vi "triquimejorado.vi"() -> ()   [LabVIEW 2021]
panel:
  out "appended array":u16[][](array[numeric])
  in  "OK Button":bool
  in  "x":bool
  in  "Ring 9":u16(ring)
  in  "Ring 8":u16(ring)
  in  "Ring 6":u16(ring)
  in  "Ring 5":u16(ring)
  in  "Ring 7":u16(ring)
  in  "Ring 4":u16(ring)
  in  "Ring 3":u16(ring)
  in  "Ring 2":u16(ring)
  in  "Ring":u16(ring)
  # "0"
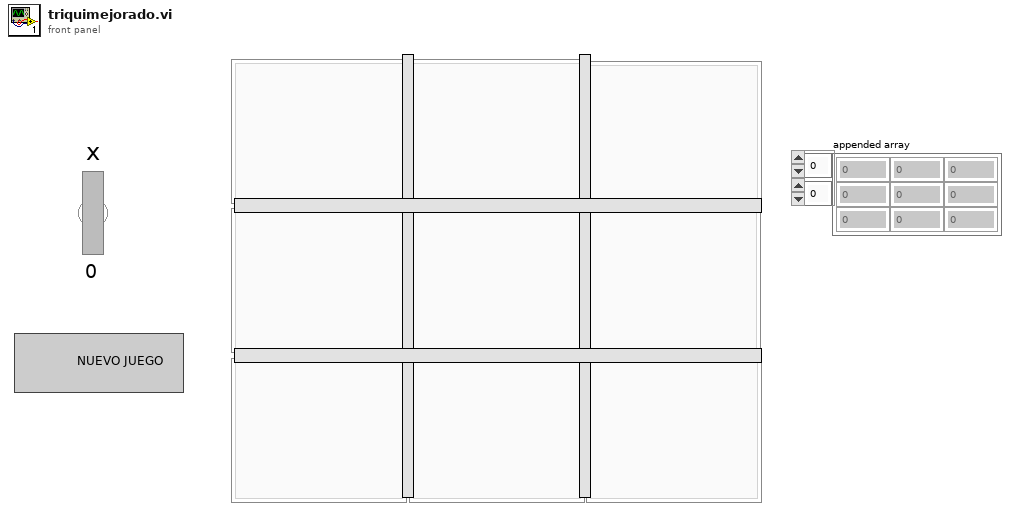
[diagram p1: front panel]
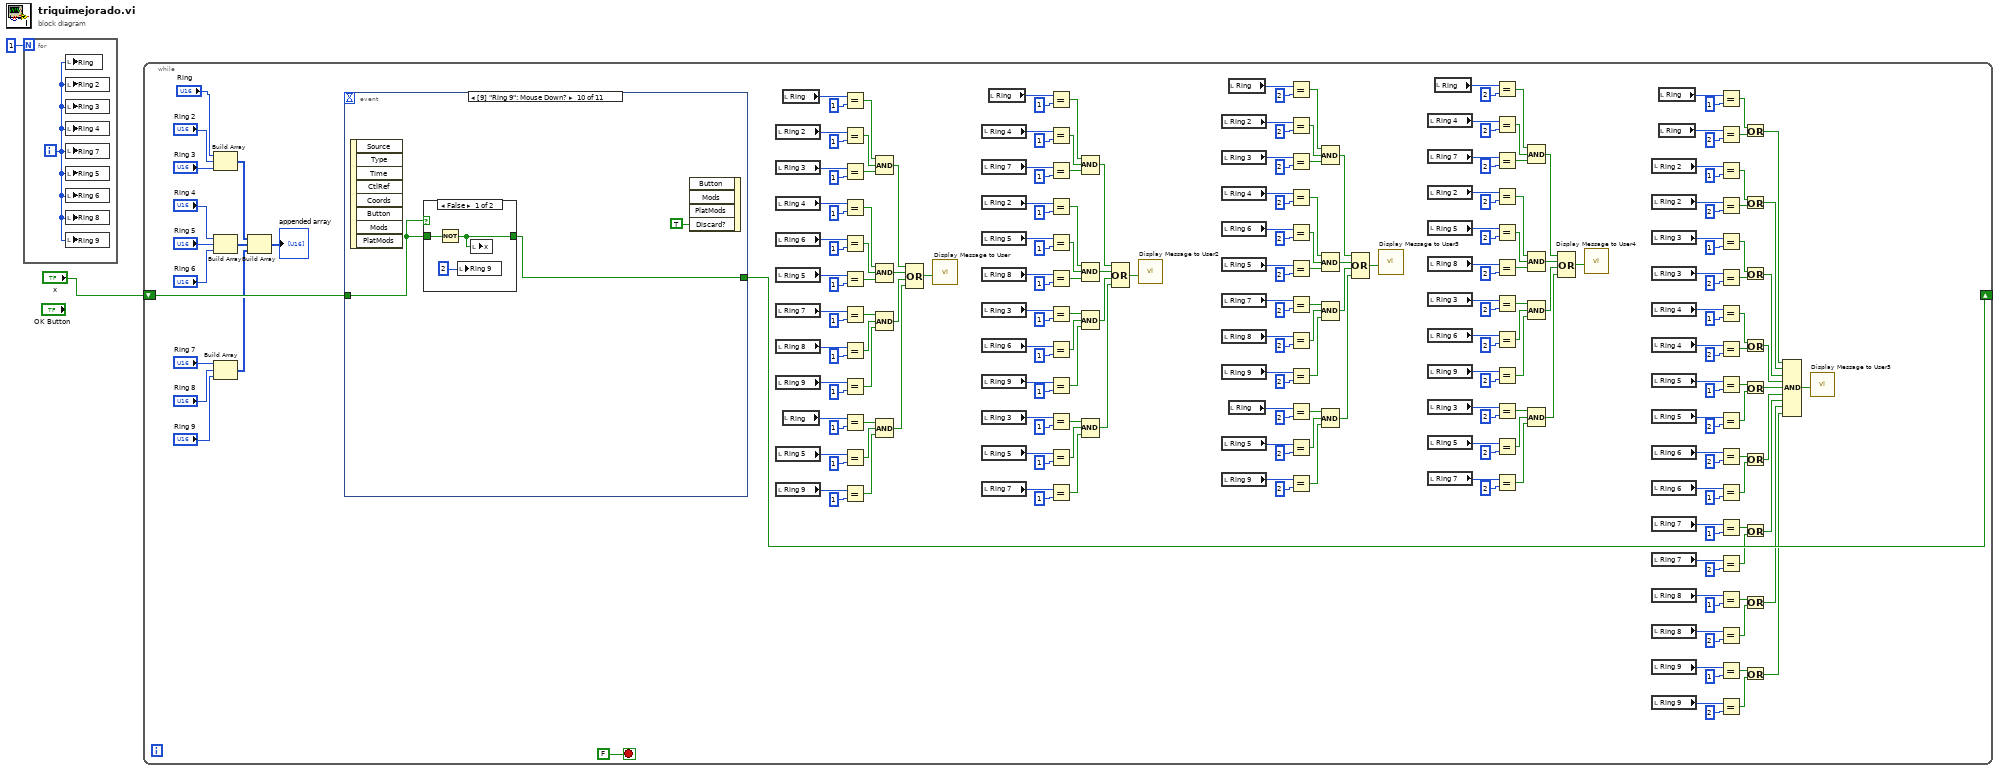
[diagram p0: block diagram]
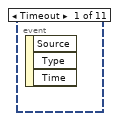
[diagram p2: hidden frame]
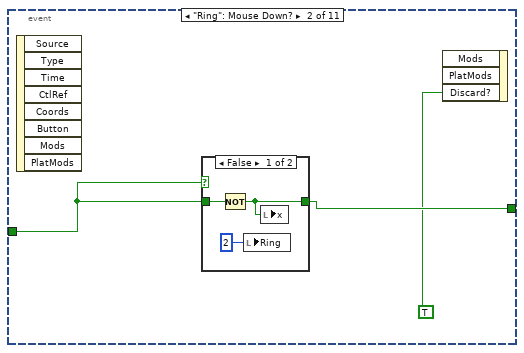
[diagram p3: hidden frame]
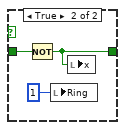
[diagram p4: hidden frame]
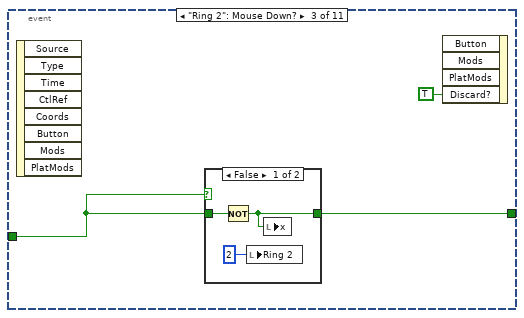
[diagram p5: hidden frame]
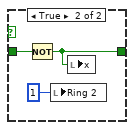
[diagram p6: hidden frame]
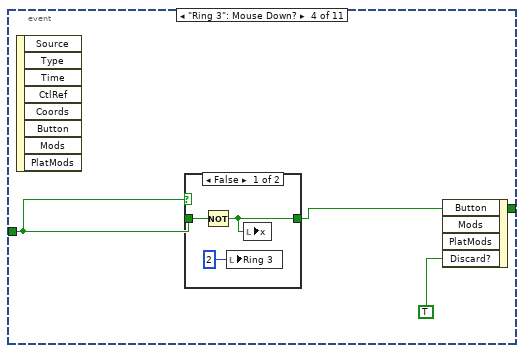
[diagram p7: hidden frame]
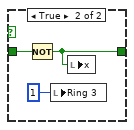
[diagram p8: hidden frame]
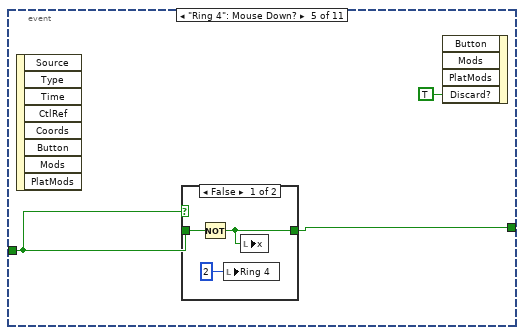
[diagram p9: hidden frame]
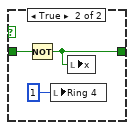
[diagram p10: hidden frame]
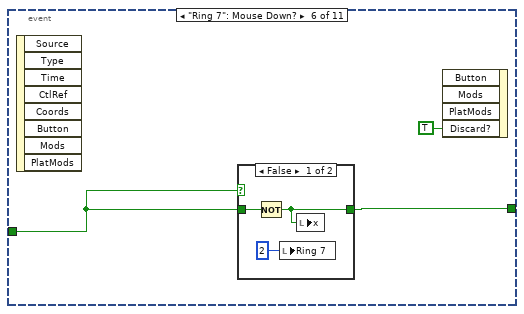
[diagram p11: hidden frame]
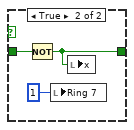
[diagram p12: hidden frame]
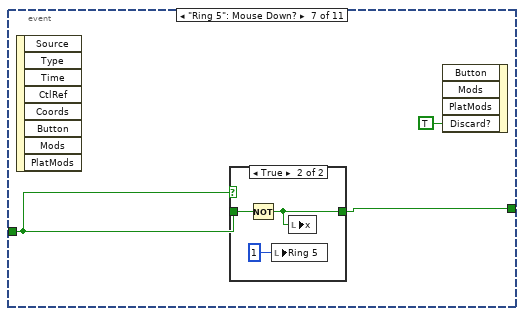
[diagram p13: hidden frame]
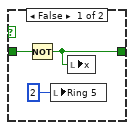
[diagram p14: hidden frame]
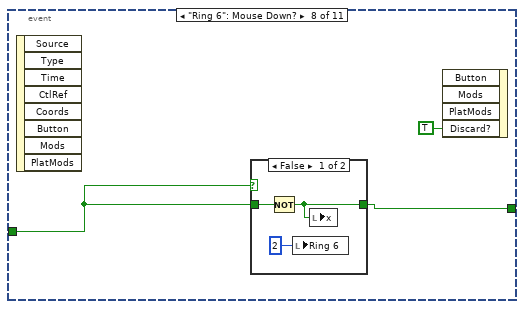
[diagram p15: hidden frame]
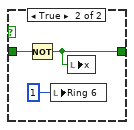
[diagram p16: hidden frame]
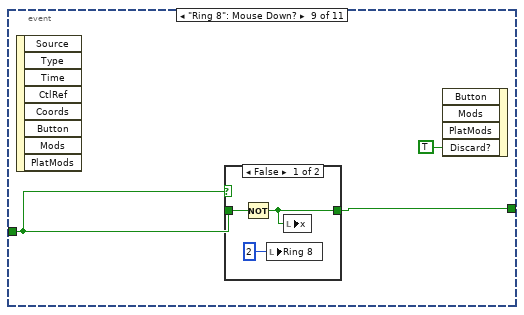
[diagram p17: hidden frame]
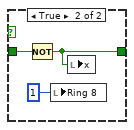
[diagram p18: hidden frame]
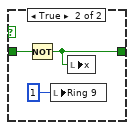
[diagram p19: hidden frame]
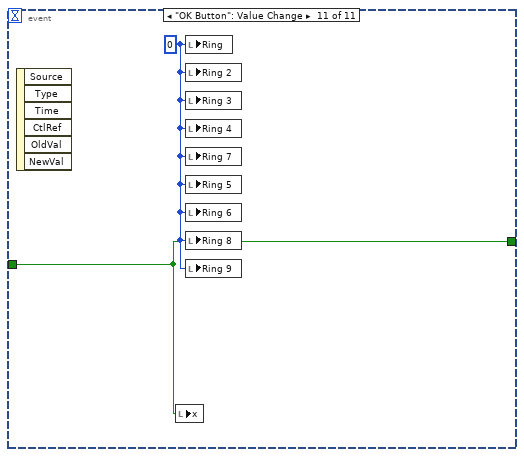
[diagram p20: hidden frame]
diagram:
  n1 = for {
    N: 1 -> [_]
    i -> [w3]
    n2 = local write "Ring"(w3) -> ()
    n3 = local write "Ring 2"(w3) -> ()
    n4 = local write "Ring 3"(w3) -> ()
    n5 = local write "Ring 4"(w3) -> ()
    n6 = local write "Ring 7"(w3) -> ()
    n7 = local write "Ring 5"(w3) -> ()
    n8 = local write "Ring 6"(w3) -> ()
    n9 = local write "Ring 8"(w3) -> ()
    n10 = local write "Ring 9"(w3) -> ()
  }
  n11 = while {
    shift-right: [w247] -> _
    shift-left: "x" -> [w246]
    stop <- FALSE stop-if-true
    n12 = Build Array("Ring", "Ring 2", "Ring 3") -> (w75:u16[])
    n13 = Build Array("Ring 4", "Ring 5", "Ring 6") -> (w74:u16[])
    n14 = Build Array("Ring 7", "Ring 8", "Ring 9") -> (w76:u16[])
    n15 = Build Array(w75, w74, w76) -> (→"appended array":u16[][])
    n16 = event shown="[9] \"Ring 9\": Mouse Down?" {
      selector: _ -> [_ _ _ _ _ _ _ _ _ _ _]
      dyn-events: _ -> [_ _ _ _ _ _ _ _ _ _ _]
      timeout: _ -> [_ _ _ _ _ _ _ _ _ _ _]
      tunnel: [_ w250 w258 w267 w276 w286 w295 w304 w312 w321 w329] -> w247
      tunnel: w246 -> [_ w248 w259 w268 w277 w285 w294 w303 w313 w322 w329]
      event Timeout {
        n17 = event-data() -> ()  [unwired: 1 in, 3 out]
      }
      event "Ring": Mouse Down? {
        n18 = event-data() -> ()  [unwired: 1 in, 8 out]
        n19 = case shown="False" w248 {
          tunnel: [w252 w255] -> w250
          tunnel: w248 -> [w251 w254]
          frame False {
            n20 = Not(x=w251) -> (.not. x?=w252:bool)
            n21 = local write "Ring"(u16 2 ("Ring")) -> ()
            n22 = local write "x"(w252) -> ()
          }
          frame True {
            n23 = Not(x=w254) -> (.not. x?=w255:bool)
            n24 = local write "Ring"(u16 1 ("Ring")) -> ()
            n25 = local write "x"(w255) -> ()
          }
        }
        n26 = event-data("Discard?"=TRUE) -> ()  [unwired: 3 in, 1 out]
      }
      event "Ring 2": Mouse Down? {
        n27 = event-data() -> ()  [unwired: 1 in, 8 out]
        n28 = case shown="False" w259 {
          tunnel: w259 -> [w261 w264]
          tunnel: [w260 w263] -> w258
          frame False {
            n29 = Not(x=w261) -> (.not. x?=w260:bool)
            n30 = local write "Ring 2"(u16 2 ("Ring 2")) -> ()
            n31 = local write "x"(w260) -> ()
          }
          frame True {
            n32 = Not(x=w264) -> (.not. x?=w263:bool)
            n33 = local write "Ring 2"(u16 1 ("Ring 2")) -> ()
            n34 = local write "x"(w263) -> ()
          }
        }
        n35 = event-data("Discard?"=TRUE) -> ()  [unwired: 4 in, 1 out]
      }
      event "Ring 3": Mouse Down? {
        n36 = event-data() -> ()  [unwired: 1 in, 8 out]
        n37 = case shown="False" w268 {
          tunnel: w268 -> [w270 w273]
          tunnel: [w269 w272] -> w267
          frame False {
            n38 = Not(x=w270) -> (.not. x?=w269:bool)
            n39 = local write "Ring 3"(u16 2 ("Ring 2")) -> ()
            n40 = local write "x"(w269) -> ()
          }
          frame True {
            n41 = Not(x=w273) -> (.not. x?=w272:bool)
            n42 = local write "Ring 3"(u16 1 ("Ring 2")) -> ()
            n43 = local write "x"(w272) -> ()
          }
        }
        n44 = event-data("Discard?"=TRUE) -> ()  [unwired: 4 in, 1 out]
      }
      event "Ring 4": Mouse Down? {
        n45 = event-data() -> ()  [unwired: 1 in, 8 out]
        n46 = case shown="False" w277 {
          tunnel: w277 -> [w279 w282]
          tunnel: [w278 w281] -> w276
          frame False {
            n47 = Not(x=w279) -> (.not. x?=w278:bool)
            n48 = local write "Ring 4"(u16 2 ("Ring 2")) -> ()
            n49 = local write "x"(w278) -> ()
          }
          frame True {
            n50 = Not(x=w282) -> (.not. x?=w281:bool)
            n51 = local write "Ring 4"(u16 1 ("Ring 2")) -> ()
            n52 = local write "x"(w281) -> ()
          }
        }
        n53 = event-data("Discard?"=TRUE) -> ()  [unwired: 4 in, 1 out]
      }
      event "Ring 7": Mouse Down? {
        n54 = event-data() -> ()  [unwired: 1 in, 8 out]
        n55 = case shown="False" w285 {
          tunnel: w285 -> [w288 w291]
          tunnel: [w287 w290] -> w286
          frame False {
            n56 = Not(x=w288) -> (.not. x?=w287:bool)
            n57 = local write "Ring 7"(u16 2 ("Ring 2")) -> ()
            n58 = local write "x"(w287) -> ()
          }
          frame True {
            n59 = Not(x=w291) -> (.not. x?=w290:bool)
            n60 = local write "Ring 7"(u16 1 ("Ring 2")) -> ()
            n61 = local write "x"(w290) -> ()
          }
        }
        n62 = event-data("Discard?"=TRUE) -> ()  [unwired: 4 in, 1 out]
      }
      event "Ring 5": Mouse Down? {
        n63 = event-data() -> ()  [unwired: 1 in, 8 out]
        n64 = case shown="True" w294 {
          tunnel: w294 -> [w297 w300]
          tunnel: [w296 w299] -> w295
          frame False {
            n65 = Not(x=w297) -> (.not. x?=w296:bool)
            n66 = local write "Ring 5"(u16 2 ("Ring 2")) -> ()
            n67 = local write "x"(w296) -> ()
          }
          frame True {
            n68 = Not(x=w300) -> (.not. x?=w299:bool)
            n69 = local write "Ring 5"(u16 1 ("Ring 2")) -> ()
            n70 = local write "x"(w299) -> ()
          }
        }
        n71 = event-data("Discard?"=TRUE) -> ()  [unwired: 4 in, 1 out]
      }
      event "Ring 6": Mouse Down? {
        n72 = event-data() -> ()  [unwired: 1 in, 8 out]
        n73 = case shown="False" w303 {
          tunnel: w303 -> [w306 w309]
          tunnel: [w305 w308] -> w304
          frame False {
            n74 = Not(x=w306) -> (.not. x?=w305:bool)
            n75 = local write "Ring 6"(u16 2 ("Ring 2")) -> ()
            n76 = local write "x"(w305) -> ()
          }
          frame True {
            n77 = Not(x=w309) -> (.not. x?=w308:bool)
            n78 = local write "Ring 6"(u16 1 ("Ring 2")) -> ()
            n79 = local write "x"(w308) -> ()
          }
        }
        n80 = event-data("Discard?"=TRUE) -> ()  [unwired: 4 in, 1 out]
      }
      event "Ring 8": Mouse Down? {
        n81 = event-data() -> ()  [unwired: 1 in, 8 out]
        n82 = case shown="False" w313 {
          tunnel: w313 -> [w315 w318]
          tunnel: [w314 w317] -> w312
          frame False {
            n83 = Not(x=w315) -> (.not. x?=w314:bool)
            n84 = local write "Ring 8"(u16 2 ("Ring 2")) -> ()
            n85 = local write "x"(w314) -> ()
          }
          frame True {
            n86 = Not(x=w318) -> (.not. x?=w317:bool)
            n87 = local write "Ring 8"(u16 1 ("Ring 2")) -> ()
            n88 = local write "x"(w317) -> ()
          }
        }
        n89 = event-data("Discard?"=TRUE) -> ()  [unwired: 4 in, 1 out]
      }
      event "Ring 9": Mouse Down? {
        n90 = event-data() -> ()  [unwired: 1 in, 8 out]
        n91 = case shown="False" w322 {
          tunnel: w322 -> [w324 w327]
          tunnel: [w323 w326] -> w321
          frame False {
            n92 = Not(x=w324) -> (.not. x?=w323:bool)
            n93 = local write "Ring 9"(u16 2 ("Ring 2")) -> ()
            n94 = local write "x"(w323) -> ()
          }
          frame True {
            n95 = Not(x=w327) -> (.not. x?=w326:bool)
            n96 = local write "Ring 9"(u16 1 ("Ring 2")) -> ()
            n97 = local write "x"(w326) -> ()
          }
        }
        n98 = event-data("Discard?"=TRUE) -> ()  [unwired: 4 in, 1 out]
      }
      event "OK Button": Value Change {
        w330 = u16 0 ("Ring")
        n99 = event-data() -> ()  [unwired: 1 in, 6 out]
        n100 = local write "x"(w329) -> ()
        n101 = local write "Ring"(w330) -> ()
        n102 = local write "Ring 2"(w330) -> ()
        n103 = local write "Ring 3"(w330) -> ()
        n104 = local write "Ring 4"(w330) -> ()
        n105 = local write "Ring 7"(w330) -> ()
        n106 = local write "Ring 5"(w330) -> ()
        n107 = local write "Ring 6"(w330) -> ()
        n108 = local write "Ring 8"(w330) -> ()
        n109 = local write "Ring 9"(w330) -> ()
      }
    }
    n110 = local read "Ring 2"() -> (w243:u16)
    n111 = local read "Ring 3"() -> (w241:u16)
    n112 = local read "Ring 4"() -> (w230:u16)
    n113 = local read "Ring 6"() -> (w229:u16)
    n114 = local read "Ring 5"() -> (w228:u16)
    n115 = local read "Ring 7"() -> (w221:u16)
    n116 = local read "Ring 8"() -> (w220:u16)
    n117 = local read "Ring 9"() -> (w219:u16)
    n118 = local read "Ring 5"() -> (w213:u16)
    n119 = local read "Ring 9"() -> (w214:u16)
    n120 = local read "Ring"() -> (w245:u16)
    n121 = local read "Ring"() -> (w212:u16)
    n122 = Equal?(x=w245, y=u16 1) -> (x = y?=w239:bool)
    n123 = Equal?(x=w243, y=u16 1) -> (x = y?=w238:bool)
    n124 = Equal?(x=w241, y=u16 1) -> (x = y?=w237:bool)
    n125 = Equal?(x=w230, y=u16 1) -> (x = y?=w234:bool)
    n126 = Equal?(x=w229, y=u16 1) -> (x = y?=w235:bool)
    n127 = Equal?(x=w228, y=u16 1) -> (x = y?=w236:bool)
    n128 = Equal?(x=w221, y=u16 1) -> (x = y?=w224:bool)
    n129 = Equal?(x=w220, y=u16 1) -> (x = y?=w223:bool)
    n130 = Equal?(x=w219, y=u16 1) -> (x = y?=w222:bool)
    n131 = Equal?(x=w212, y=u16 1) -> (x = y?=w209:bool)
    n132 = Equal?(x=w213, y=u16 1) -> (x = y?=w210:bool)
    n133 = Equal?(x=w214, y=u16 1) -> (x = y?=w211:bool)
    n134 = Compound Arithmetic op=AND(w239, w238, w237) -> (w218:bool)
    n135 = Compound Arithmetic op=AND(w234, w235, w236) -> (w217:bool)
    n136 = Compound Arithmetic op=AND(w224, w223, w222) -> (w216:bool)
    n137 = Compound Arithmetic op=AND(w209, w210, w211) -> (w205:bool)
    n138 = Compound Arithmetic op=OR(w218, w217, w216, w205) -> (w215:bool)
    n139 = call "Display Message to User"("Enable"=w215) -> ()  [unwired: 9 in, 2 out]
    n140 = local read "Ring 4"() -> (w166:u16)
    n141 = local read "Ring 7"() -> (w168:u16)
    n142 = local read "Ring 2"() -> (w179:u16)
    n143 = local read "Ring 5"() -> (w180:u16)
    n144 = local read "Ring 8"() -> (w181:u16)
    n145 = local read "Ring 3"() -> (w188:u16)
    n146 = local read "Ring 6"() -> (w189:u16)
    n147 = local read "Ring 9"() -> (w190:u16)
    n148 = local read "Ring 3"() -> (w197:u16)
    n149 = local read "Ring 5"() -> (w196:u16)
    n150 = local read "Ring 7"() -> (w195:u16)
    n151 = local read "Ring"() -> (w164:u16)
    n152 = Equal?(x=w164, y=u16 1) -> (x = y?=w170:bool)
    n153 = Equal?(x=w166, y=u16 1) -> (x = y?=w171:bool)
    n154 = Equal?(x=w168, y=u16 1) -> (x = y?=w172:bool)
    n155 = Equal?(x=w179, y=u16 1) -> (x = y?=w175:bool)
    n156 = Equal?(x=w180, y=u16 1) -> (x = y?=w174:bool)
    n157 = Equal?(x=w181, y=u16 1) -> (x = y?=w173:bool)
    n158 = Equal?(x=w188, y=u16 1) -> (x = y?=w185:bool)
    n159 = Equal?(x=w189, y=u16 1) -> (x = y?=w186:bool)
    n160 = Equal?(x=w190, y=u16 1) -> (x = y?=w187:bool)
    n161 = Equal?(x=w197, y=u16 1) -> (x = y?=w200:bool)
    n162 = Equal?(x=w196, y=u16 1) -> (x = y?=w199:bool)
    n163 = Equal?(x=w195, y=u16 1) -> (x = y?=w198:bool)
    n164 = Compound Arithmetic op=AND(w170, w171, w172) -> (w191:bool)
    n165 = Compound Arithmetic op=AND(w175, w174, w173) -> (w192:bool)
    n166 = Compound Arithmetic op=AND(w185, w186, w187) -> (w193:bool)
    n167 = Compound Arithmetic op=AND(w200, w199, w198) -> (w204:bool)
    n168 = Compound Arithmetic op=OR(w191, w192, w193, w204) -> (w194:bool)
    n169 = call "Display Message to User2"("Enable"=w194) -> ()  [unwired: 9 in, 2 out]
    n170 = local read "Ring 2"() -> (w84:u16)
    n171 = local read "Ring 3"() -> (w86:u16)
    n172 = local read "Ring 4"() -> (w97:u16)
    n173 = local read "Ring 6"() -> (w98:u16)
    n174 = local read "Ring 5"() -> (w99:u16)
    n175 = local read "Ring 7"() -> (w106:u16)
    n176 = local read "Ring 8"() -> (w107:u16)
    n177 = local read "Ring 9"() -> (w108:u16)
    n178 = local read "Ring 5"() -> (w114:u16)
    n179 = local read "Ring 9"() -> (w113:u16)
    n180 = local read "Ring"() -> (w82:u16)
    n181 = local read "Ring"() -> (w115:u16)
    n182 = Equal?(x=w82, y=u16 2) -> (x = y?=w88:bool)
    n183 = Equal?(x=w84, y=u16 2) -> (x = y?=w89:bool)
    n184 = Equal?(x=w86, y=u16 2) -> (x = y?=w90:bool)
    n185 = Equal?(x=w97, y=u16 2) -> (x = y?=w93:bool)
    n186 = Equal?(x=w98, y=u16 2) -> (x = y?=w92:bool)
    n187 = Equal?(x=w99, y=u16 2) -> (x = y?=w91:bool)
    n188 = Equal?(x=w106, y=u16 2) -> (x = y?=w103:bool)
    n189 = Equal?(x=w107, y=u16 2) -> (x = y?=w104:bool)
    n190 = Equal?(x=w108, y=u16 2) -> (x = y?=w105:bool)
    n191 = Equal?(x=w115, y=u16 2) -> (x = y?=w118:bool)
    n192 = Equal?(x=w114, y=u16 2) -> (x = y?=w117:bool)
    n193 = Equal?(x=w113, y=u16 2) -> (x = y?=w116:bool)
    n194 = Compound Arithmetic op=AND(w88, w89, w90) -> (w109:bool)
    n195 = Compound Arithmetic op=AND(w93, w92, w91) -> (w110:bool)
    n196 = Compound Arithmetic op=AND(w103, w104, w105) -> (w111:bool)
    n197 = Compound Arithmetic op=AND(w118, w117, w116) -> (w122:bool)
    n198 = Compound Arithmetic op=OR(w109, w110, w111, w122) -> (w112:bool)
    n199 = call "Display Message to User3"("Enable"=w112) -> ()  [unwired: 9 in, 2 out]
    n200 = local read "Ring 4"() -> (w161:u16)
    n201 = local read "Ring 7"() -> (w159:u16)
    n202 = local read "Ring 2"() -> (w148:u16)
    n203 = local read "Ring 5"() -> (w147:u16)
    n204 = local read "Ring 8"() -> (w146:u16)
    n205 = local read "Ring 3"() -> (w139:u16)
    n206 = local read "Ring 6"() -> (w138:u16)
    n207 = local read "Ring 9"() -> (w137:u16)
    n208 = local read "Ring 3"() -> (w130:u16)
    n209 = local read "Ring 5"() -> (w131:u16)
    n210 = local read "Ring 7"() -> (w132:u16)
    n211 = local read "Ring"() -> (w163:u16)
    n212 = Equal?(x=w163, y=u16 2) -> (x = y?=w157:bool)
    n213 = Equal?(x=w161, y=u16 2) -> (x = y?=w156:bool)
    n214 = Equal?(x=w159, y=u16 2) -> (x = y?=w155:bool)
    n215 = Equal?(x=w148, y=u16 2) -> (x = y?=w152:bool)
    n216 = Equal?(x=w147, y=u16 2) -> (x = y?=w153:bool)
    n217 = Equal?(x=w146, y=u16 2) -> (x = y?=w154:bool)
    n218 = Equal?(x=w139, y=u16 2) -> (x = y?=w142:bool)
    n219 = Equal?(x=w138, y=u16 2) -> (x = y?=w141:bool)
    n220 = Equal?(x=w137, y=u16 2) -> (x = y?=w140:bool)
    n221 = Equal?(x=w130, y=u16 2) -> (x = y?=w127:bool)
    n222 = Equal?(x=w131, y=u16 2) -> (x = y?=w128:bool)
    n223 = Equal?(x=w132, y=u16 2) -> (x = y?=w129:bool)
    n224 = Compound Arithmetic op=AND(w157, w156, w155) -> (w136:bool)
    n225 = Compound Arithmetic op=AND(w152, w153, w154) -> (w135:bool)
    n226 = Compound Arithmetic op=AND(w142, w141, w140) -> (w134:bool)
    n227 = Compound Arithmetic op=AND(w127, w128, w129) -> (w123:bool)
    n228 = Compound Arithmetic op=OR(w136, w135, w134, w123) -> (w133:bool)
    n229 = call "Display Message to User4"("Enable"=w133) -> ()  [unwired: 9 in, 2 out]
    n230 = local read "Ring 2"() -> (w60:u16)
    n231 = local read "Ring 2"() -> (w63:u16)
    n232 = local read "Ring 3"() -> (w59:u16)
    n233 = local read "Ring 3"() -> (w56:u16)
    n234 = local read "Ring 4"() -> (w52:u16)
    n235 = local read "Ring 4"() -> (w55:u16)
    n236 = local read "Ring 5"() -> (w51:u16)
    n237 = local read "Ring 5"() -> (w48:u16)
    n238 = local read "Ring 6"() -> (w47:u16)
    n239 = local read "Ring 6"() -> (w44:u16)
    n240 = local read "Ring 7"() -> (w43:u16)
    n241 = local read "Ring 7"() -> (w40:u16)
    n242 = local read "Ring 8"() -> (w36:u16)
    n243 = local read "Ring 8"() -> (w39:u16)
    n244 = local read "Ring 9"() -> (w35:u16)
    n245 = local read "Ring 9"() -> (w32:u16)
    n246 = local read "Ring"() -> (w67:u16)
    n247 = local read "Ring"() -> (w64:u16)
    n248 = Equal?(x=w67, y=u16 1) -> (x = y?=w31:bool)
    n249 = Equal?(x=w64, y=u16 2) -> (x = y?=w30:bool)
    n250 = Equal?(x=w60, y=u16 1) -> (x = y?=w29:bool)
    n251 = Equal?(x=w63, y=u16 2) -> (x = y?=w28:bool)
    n252 = Equal?(x=w59, y=u16 1) -> (x = y?=w25:bool)
    n253 = Equal?(x=w56, y=u16 2) -> (x = y?=w24:bool)
    n254 = Equal?(x=w52, y=u16 1) -> (x = y?=w23:bool)
    n255 = Equal?(x=w55, y=u16 2) -> (x = y?=w22:bool)
    n256 = Equal?(x=w51, y=u16 1) -> (x = y?=w21:bool)
    n257 = Equal?(x=w48, y=u16 2) -> (x = y?=w20:bool)
    n258 = Equal?(x=w47, y=u16 2) -> (x = y?=w19:bool)
    n259 = Equal?(x=w44, y=u16 1) -> (x = y?=w27:bool)
    n260 = Equal?(x=w43, y=u16 1) -> (x = y?=w18:bool)
    n261 = Equal?(x=w40, y=u16 2) -> (x = y?=w26:bool)
    n262 = Equal?(x=w36, y=u16 1) -> (x = y?=w17:bool)
    n263 = Equal?(x=w39, y=u16 2) -> (x = y?=w16:bool)
    n264 = Equal?(x=w35, y=u16 1) -> (x = y?=w15:bool)
    n265 = Equal?(x=w32, y=u16 2) -> (x = y?=w14:bool)
    n266 = Or(x=w31, y=w30) -> (x .or. y?=w13:bool)
    n267 = Or(x=w29, y=w28) -> (x .or. y?=w12:bool)
    n268 = Or(x=w25, y=w24) -> (x .or. y?=w11:bool)
    n269 = Or(x=w23, y=w22) -> (x .or. y?=w10:bool)
    n270 = Or(x=w21, y=w20) -> (x .or. y?=w9:bool)
    n271 = Or(x=w19, y=w27) -> (x .or. y?=w8:bool)
    n272 = Or(x=w18, y=w26) -> (x .or. y?=w7:bool)
    n273 = Or(x=w17, y=w16) -> (x .or. y?=w6:bool)
    n274 = Or(x=w15, y=w14) -> (x .or. y?=w5:bool)
    n275 = Compound Arithmetic op=AND(w13, w12, w11, w10, w9, w8, w7, w6, w5) -> (w4:bool)
    n276 = call "Display Message to User5"("Enable"=w4) -> ()  [unwired: 9 in, 2 out]
  }
